vi "MDAQ_CVPlotHelper.vi"(8 "Amplitude Plot":refnum<vi>, 9 "Normalised":bool, 10 "Input Cluster":T1 {"CV"."Temperature Array" scale=0.0..100.0}, 11 "XY Graph ref":refnum<vi>) -> ()   [LabVIEW 2021]
uses:
  GUI_Def.ctl
  Mode_Enum.ctl
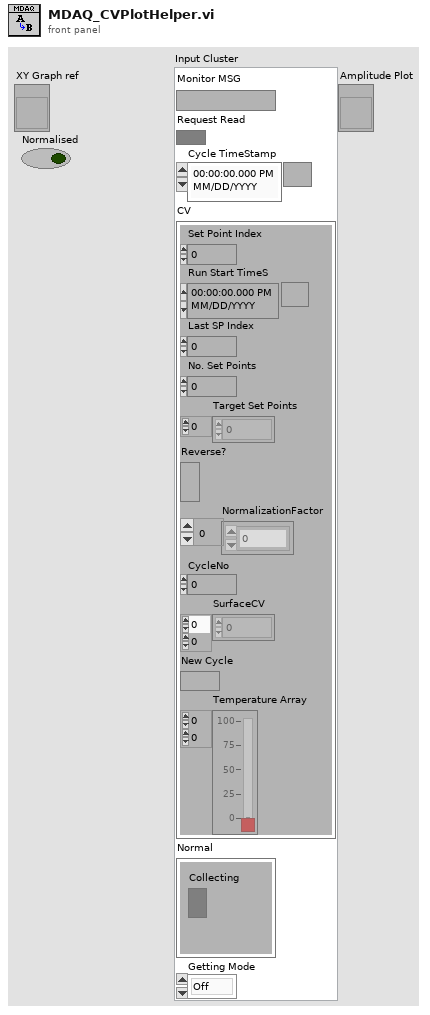
[diagram p1: front panel]
types:
  T1 = typedef "GUI_Def.ctl" = cluster{"Monitor MSG":string, "Request Read":bool, "Cycle TimeStamp":timestamp, "CV":cluster{"Set Point Index":u32, "Run Start TimeS":timestamp, "Last SP Index":u32, "No. Set Points":u32, "Target Set Points":i32[], "Reverse?":bool, "NormalizationFactor":i32[], "CycleNo":i32, "SurfaceCV":dbl[][], "New Cycle":bool, "Temperature Array":dbl[][]}, "Normal":cluster{"Collecting":bool}, "Getting Mode":T2}
  T2 = typedef "Mode_Enum.ctl" = enum16{"Off", "Normal", "CV+Temp", "CV"}
  T3 = cluster{"SetPointArray":cluster{timestamp, dbl}[]}[]
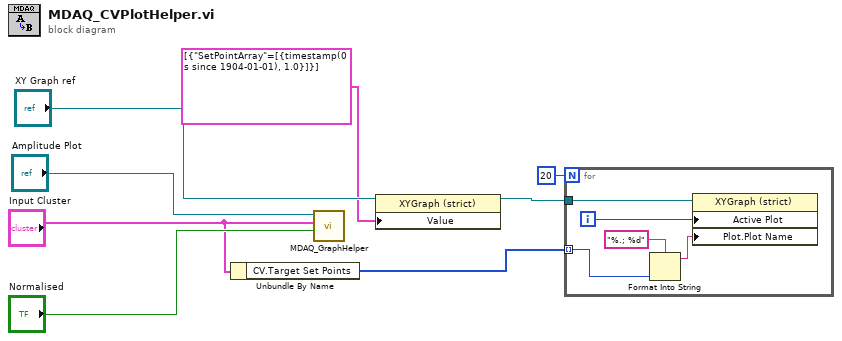
[diagram p0: block diagram]
diagram:
  n1 = Unbundle By Name("Input Cluster") -> ("CV.Target Set Points"=w5:i32[])
  n2 = call "MDAQ_GraphHelper.vi"("Normalised"="Normalised", "Input Cluster"="Input Cluster", "Amplitude Plot"="Amplitude Plot") -> ()  [unwired: 6 in, 3 out]
  n3 = property class="XYGraph (strict)"(reference="XY Graph ref", "Value"=T3 [{"SetPointArray"=[{timestamp(0 s since 1904-01-01), 1.0}]}]) -> (reference out=w4:refnum<vi>)  [unwired: 1 in, 1 out]
  n4 = for {
    N: 20 -> [_]
    tunnel: w5 -> [w11] mode=indexing
    tunnel: w4 -> [w13]
    i -> [w12]
    n5 = Format Into String(format string="%.; %d", w11) -> (resulting string=w9:string)  [unwired: 2 in, 1 out]
    n6 = property class="XYGraph (strict)"(reference=w13, "Active Plot"=w12, "Plot.Plot Name"=w9) -> ()  [unwired: 1 in, 2 out]
  }
